vi "CRC_16CITT_B.vi"(6 "Error In":errorcluster, 7 "DATA PACKET":string) -> (0 "Error Out":errorcluster, 1 "DATA PACKET+CRC":string, 2 "CRC out":u16 format="%x")   [LabVIEW 2019]
doc: "Данная VI предназначена для расчета CRC-16CITT, которая используется для стандарта ISO/IEC 14443 Type B и ISO/IEC 15693."
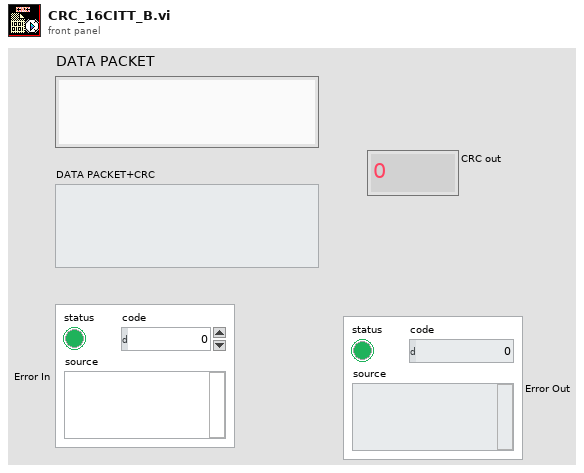
[diagram p1: front panel]
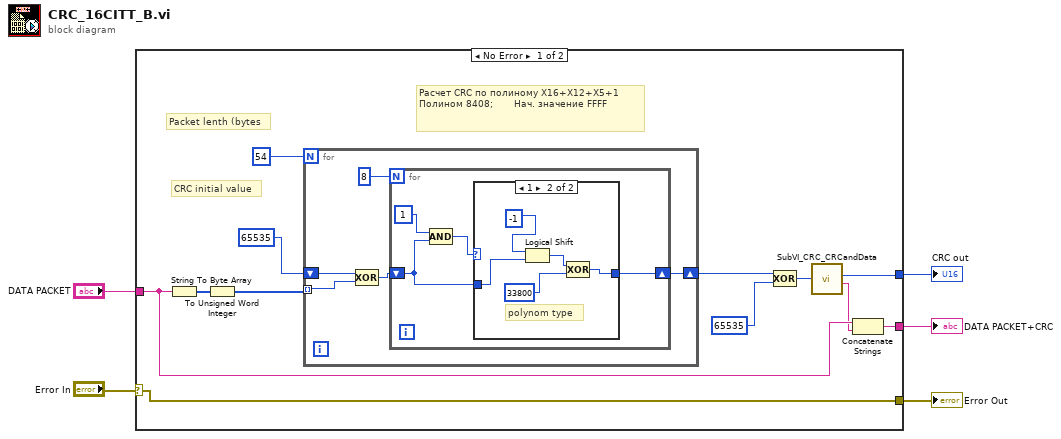
[diagram p0: block diagram]
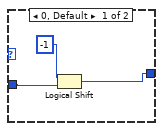
[diagram p2: hidden frame]
diagram:
  n1 = case shown="No Error" "Error In" {
    selector: "Error In" -> [w14 w36]
    tunnel: [w12 _] -> w5
    tunnel: "DATA PACKET" -> [w16 w35]
    tunnel: [w15 w35] -> w3
    tunnel: [w14 w36] -> w1
    frame No Error {
      # "Packet lenth (bytes"
      # "CRC initial value"
      # "Расчет CRC по полиному X16+X12+X5+1\nПолином 8408;       Нач. значение FFFF"
      n2 = String To Byte Array(string=w16) -> (unsigned byte array=w17:u8[])
      n3 = To Unsigned Word Integer(number=w17) -> (unsigned 16bit integer=w7:u16[])
      n4 = for {
        N: 54 -> [_]
        shift-right: [w19] -> w11
        shift-left: u16 65535 -> [w20]
        tunnel: w7 -> [w18] mode=indexing
        n5 = Compound Arithmetic op=XOR(w20, w18) -> (w21:u32)
        n6 = for {
          N: 8 -> [_]
          shift-right: [w25] -> w19
          shift-left: w21 -> [w24]
          n7 = Compound Arithmetic op=AND(u16 1, w24) -> (w23:u32)
          n8 = case shown="1" w23 {
            tunnel: [w28 w33] -> w25
            tunnel: w24 -> [w27 w30]
            frame 0, Default {
              n9 = Logical Shift(y=i16 -1, x=w27) -> (x << y=w28:u32)
            }
            frame 1 {
              # "polynom type"
              n10 = Logical Shift(y=i16 -1, x=w30) -> (x << y=w32:u32)
              n11 = Compound Arithmetic op=XOR(w32, u32 33800) -> (w33:u32)
            }
          }
        }
      }
      n12 = Compound Arithmetic op=XOR(w11, u16 65535) -> (w6:u32)
      n13 = call "SubVI_CRC_CRCandData.vi"("CRC in"=w6) -> ("CRC out(str)"=w13:string, "CRC out"=w12:u32)  [unwired: 8 in, 1 out]
      n14 = Concatenate Strings(w16, w13) -> (w15:string)
    }
    frame Error {
    }
  }
  "CRC out" <- w5
  "DATA PACKET+CRC" <- w3
  "Error Out" <- w1
